vi "4.3 CSM API String to Complex Numeric.vi"() -> ()   [LabVIEW 2017]
doc: "#### Overview\n\nDemonstrates API String support for complex numbers.\n\n#### Introduction\n\nAPI String supports complex numeric types. The format `a+bi` or `a-bi` represents a complex number, where `a` and `b` support all floating-point number expressions. The following are special cases:\n\n- An empty string converts to the prototype input value.\n- Tag:Value pairs can be parsed correctly. Tags are used only for readability and are ignored during the conversion process."
uses:
  f785d4d3-8e04-444c-8686-395012b63e33.vi
  6393c400-d1b7-4bb3-ab09-ecdbb14d8da8.vi
  ab096776-77d1-4891-b511-596120e5d7ef.vi
  0d96a7d9-ab10-448a-a9e1-40fb3bc0a402.vi
  d283d1cd-c69a-460b-b9e1-5e6c5918bb0a.vi
  97404767-118d-4f17-a2cf-1a1e5ca792b6.vi
  e575b998-367e-45b1-a456-a7b16d807cfe.vi
  c14d9f91-0602-4742-b6ef-35b5d331e3c1.vi
  f31c6302-f387-42c0-bfe2-0dea07b0aa72.vi
  cc2e84e5-a16f-4950-8d7e-5da6284e6cd8.vi
  87c63c12-d86a-4cfe-9a3b-3c80bf3e3b10.vi
  17a11460-8ac8-49ec-8a1c-4dab3b245dba.vi
  c6bb5578-7201-4a47-ae92-729fdb04bd81.vi
  b94477e1-b73a-4212-b7e2-84d28cf02f89.vi
  ca7e4b17-9ac4-4354-96d4-ac10cebb30b0.vi
  61d809a6-7a3d-44c9-89c7-b5bc536e2550.vi
  2c23c391-0876-4e17-a5de-fea836daf041.vi
  75b8f0c0-380c-46f6-9c6b-6f0a315b0ea0.vi
  addons/API-String-Arugments-Support/_Support/Data To API String Arguments.vi
  addons/API-String-Arugments-Support/_Support/Convert API String Arguments to Data(variant).vi
panel:
  out "x 9":dbl=-123.0
  out "y 9":dbl=123.0
  out "String 9":string="-123 +123i"
  out "x + iy 9":cdb=-123.0+123.0i
  out "x 8":dbl=-123000000000000.0
  out "y 8":dbl=-1.2299999999999999e-06
  out "String 8":string="-123T -1.23ui"
  out "x + iy 8":cdb=-123000000000000.0-1.23e-06i
  out "x 7":dbl=-123.0
  out "y 7":dbl=-123.0
  out "String 7":string="-123 -123i"
  out "x + iy 7":cdb=-123.0-123.0i
  out "x 6":dbl=123.0
  out "y 6":dbl=-123.0
  out "String 6":string="123 -123i"
  out "x + iy 6":cdb=123.0-123.0i
  out "x 5":dbl
  out "y 5":dbl=-123.0
  out "String 5":string="0 -123i"
  out "x + iy 5":cdb=0.0-123.0i
  out "x 4":dbl
  out "y 4":dbl=123.0
  out "String 4":string="0 +123i"
  out "x + iy 4":cdb=0.0+123.0i
  out "x 3":dbl=-123.0
  out "y 3":dbl
  out "String 3":string="-123 +0i"
  out "x + iy 3":cdb=-123.0+0.0i
  out "x 2":dbl=123.0
  out "y 2":dbl
  out "String 2":string="123 +0i"
  out "x + iy 2":cdb=123.0+0.0i
  out "x + iy":cdb
  out "String":string="0 +0i"
  out "y":dbl
  out "x":dbl
  # "#CSM-Example Overview\n\nDemonstrates API String support for complex numbers."
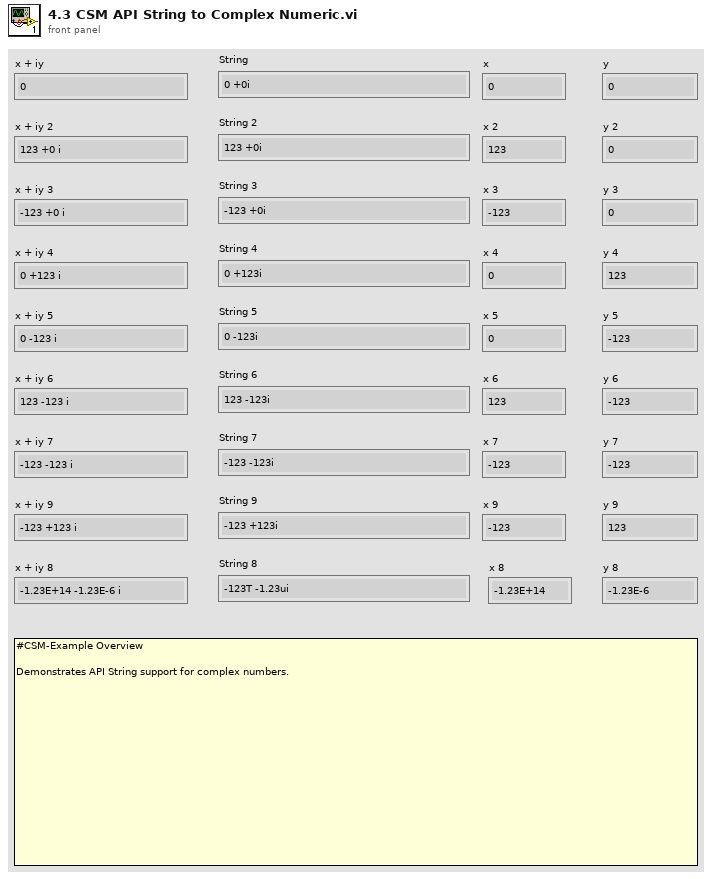
[diagram p1: front panel]
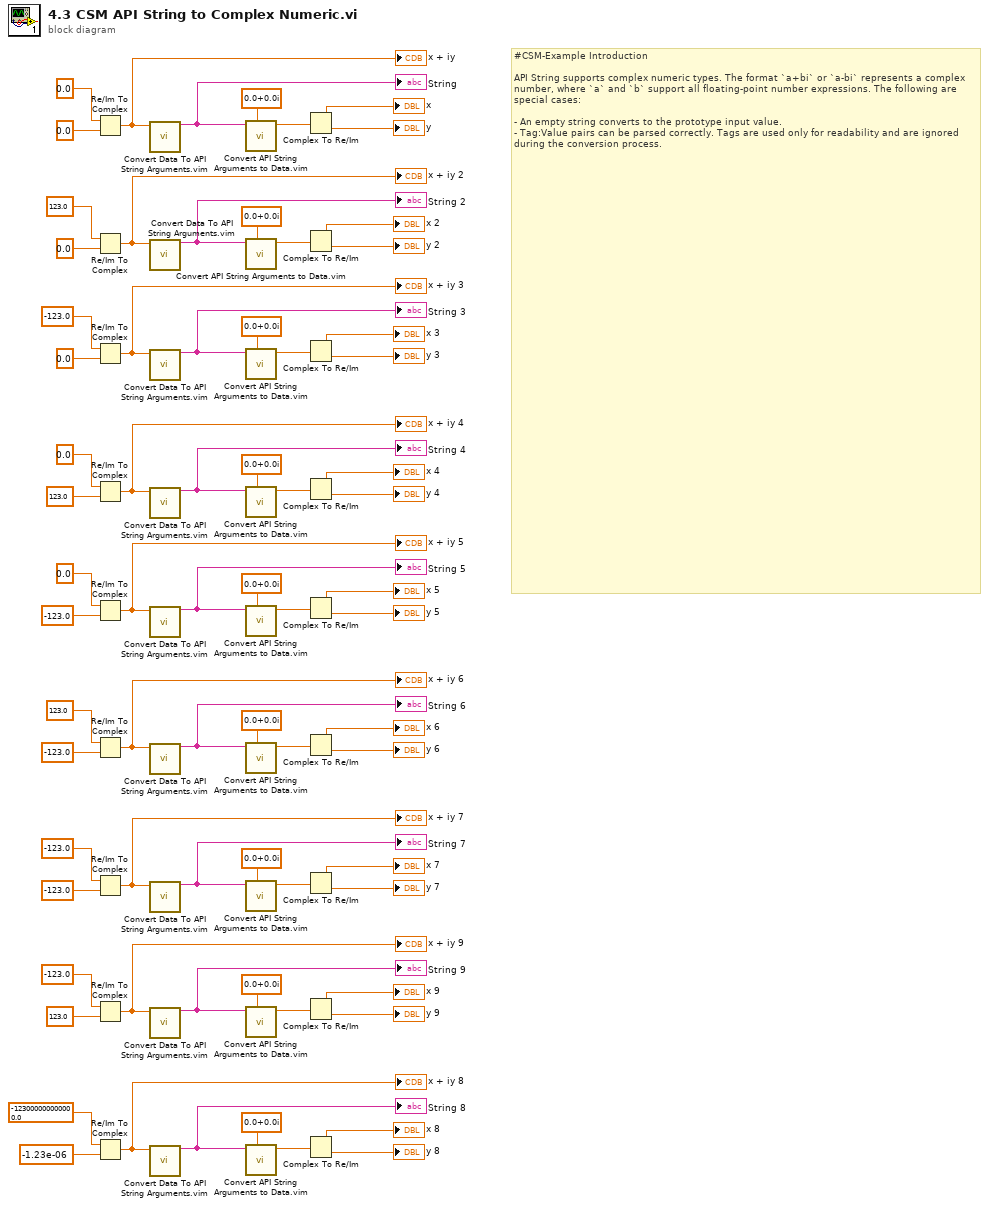
[diagram p0: block diagram]
diagram:
  # "#CSM-Example Introduction\n\nAPI String supports complex numeric types. The format `a+bi` or `a-bi` represents a complex number, where `a` and `b` support all floating-point number expressions. The following are special cases:\n\n- An empty string converts to the prototype input value.\n- Tag:Value pairs can be parsed correctly. Tags are used only for readability and are ignored during the conversion process."
  n1 = Re/Im To Complex(1:0.0 ("y"), 2:0.0 ("x")) -> (0:w71:cdb)
  "x + iy" <- w71
  n2 = Re/Im To Complex(1:0.0 ("y"), 2:123.0 ("x")) -> (0:w58:cdb)
  "x + iy 2" <- w58
  n3 = Re/Im To Complex(1:0.0 ("y"), 2:-123.0 ("x")) -> (0:w55:cdb)
  "x + iy 3" <- w55
  n4 = Re/Im To Complex(1:123.0 ("y"), 2:0.0 ("x")) -> (0:w42:cdb)
  "x + iy 4" <- w42
  n5 = Re/Im To Complex(1:-123.0 ("y"), 2:0.0 ("x")) -> (0:w39:cdb)
  "x + iy 5" <- w39
  n6 = Re/Im To Complex(1:-123.0 ("y"), 2:123.0 ("x")) -> (0:w26:cdb)
  "x + iy 6" <- w26
  n7 = Re/Im To Complex(1:-123.0 ("y"), 2:-123.0 ("x")) -> (0:w23:cdb)
  "x + iy 7" <- w23
  n8 = Re/Im To Complex(1:123.0 ("y"), 2:-123.0 ("x")) -> (0:w7:cdb)
  "x + iy 9" <- w7
  n9 = Re/Im To Complex(1:-1.23e-06 ("y"), 2:-123000000000000.0 ("x")) -> (0:w10:cdb)
  "x + iy 8" <- w10
  n10 = call "Convert Data To API String Arguments.vim"("Data"=w71) -> ("API String"=w72:string)  [unwired: 7 in, 1 out]
  "String" <- w72
  n11 = call "Convert Data To API String Arguments.vim"("Data"=w58) -> ("API String"=w57:string)  [unwired: 7 in, 1 out]
  "String 2" <- w57
  n12 = call "Convert Data To API String Arguments.vim"("Data"=w55) -> ("API String"=w56:string)  [unwired: 7 in, 1 out]
  "String 3" <- w56
  n13 = call "Convert Data To API String Arguments.vim"("Data"=w42) -> ("API String"=w41:string)  [unwired: 7 in, 1 out]
  "String 4" <- w41
  n14 = call "Convert Data To API String Arguments.vim"("Data"=w39) -> ("API String"=w40:string)  [unwired: 7 in, 1 out]
  "String 5" <- w40
  n15 = call "Convert Data To API String Arguments.vim"("Data"=w26) -> ("API String"=w25:string)  [unwired: 7 in, 1 out]
  "String 6" <- w25
  n16 = call "Convert Data To API String Arguments.vim"("Data"=w23) -> ("API String"=w24:string)  [unwired: 7 in, 1 out]
  "String 7" <- w24
  n17 = call "Convert Data To API String Arguments.vim"("Data"=w7) -> ("API String"=w8:string)  [unwired: 7 in, 1 out]
  "String 9" <- w8
  n18 = call "Convert Data To API String Arguments.vim"("Data"=w10) -> ("API String"=w9:string)  [unwired: 7 in, 1 out]
  "String 8" <- w9
  n19 = call "Convert API String Arguments to Data.vim"("Reference Type"=cdb 0.0+0.0i ("x + iy"), "API String"=w72) -> ("Data"=w68:cdb)  [unwired: 6 in, 1 out]
  n20 = call "Convert API String Arguments to Data.vim"("Reference Type"=cdb 0.0+0.0i ("x + iy"), "API String"=w57) -> ("Data"=w61:cdb)  [unwired: 6 in, 1 out]
  n21 = call "Convert API String Arguments to Data.vim"("Reference Type"=cdb 0.0+0.0i ("x + iy"), "API String"=w56) -> ("Data"=w52:cdb)  [unwired: 6 in, 1 out]
  n22 = call "Convert API String Arguments to Data.vim"("Reference Type"=cdb 0.0+0.0i ("x + iy"), "API String"=w41) -> ("Data"=w45:cdb)  [unwired: 6 in, 1 out]
  n23 = call "Convert API String Arguments to Data.vim"("Reference Type"=cdb 0.0+0.0i ("x + iy"), "API String"=w40) -> ("Data"=w36:cdb)  [unwired: 6 in, 1 out]
  n24 = call "Convert API String Arguments to Data.vim"("Reference Type"=cdb 0.0+0.0i ("x + iy"), "API String"=w25) -> ("Data"=w29:cdb)  [unwired: 6 in, 1 out]
  n25 = call "Convert API String Arguments to Data.vim"("Reference Type"=cdb 0.0+0.0i ("x + iy"), "API String"=w24) -> ("Data"=w20:cdb)  [unwired: 6 in, 1 out]
  n26 = call "Convert API String Arguments to Data.vim"("Reference Type"=cdb 0.0+0.0i ("x + iy"), "API String"=w8) -> ("Data"=w4:cdb)  [unwired: 6 in, 1 out]
  n27 = call "Convert API String Arguments to Data.vim"("Reference Type"=cdb 0.0+0.0i ("x + iy"), "API String"=w9) -> ("Data"=w13:cdb)  [unwired: 6 in, 1 out]
  n28 = Complex To Re/Im(x + iy=w68) -> (x=→"x":dbl, y=→"y":dbl)
  n29 = Complex To Re/Im(x + iy=w61) -> (x=→"x 2":dbl, y=→"y 2":dbl)
  n30 = Complex To Re/Im(x + iy=w52) -> (x=→"x 3":dbl, y=→"y 3":dbl)
  n31 = Complex To Re/Im(x + iy=w45) -> (x=→"x 4":dbl, y=→"y 4":dbl)
  n32 = Complex To Re/Im(x + iy=w36) -> (x=→"x 5":dbl, y=→"y 5":dbl)
  n33 = Complex To Re/Im(x + iy=w29) -> (x=→"x 6":dbl, y=→"y 6":dbl)
  n34 = Complex To Re/Im(x + iy=w20) -> (x=→"x 7":dbl, y=→"y 7":dbl)
  n35 = Complex To Re/Im(x + iy=w4) -> (x=→"x 9":dbl, y=→"y 9":dbl)
  n36 = Complex To Re/Im(x + iy=w13) -> (x=→"x 8":dbl, y=→"y 8":dbl)
